vi "SG_changeFrequency.vi"(7 "MHz":i32, 8 "error in":errorcluster, 11 "VISA in":refnum<visa-resource-name>) -> (0 "error out":errorcluster, 2 "SG_Resp":string, 3 "VISA out":refnum<visa-resource-name>)   [LabVIEW 2023, in "Keysight.lvlib"]
uses:
  Keysight.lvlib
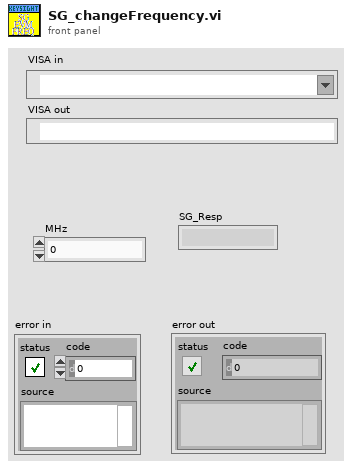
[diagram p1: front panel]
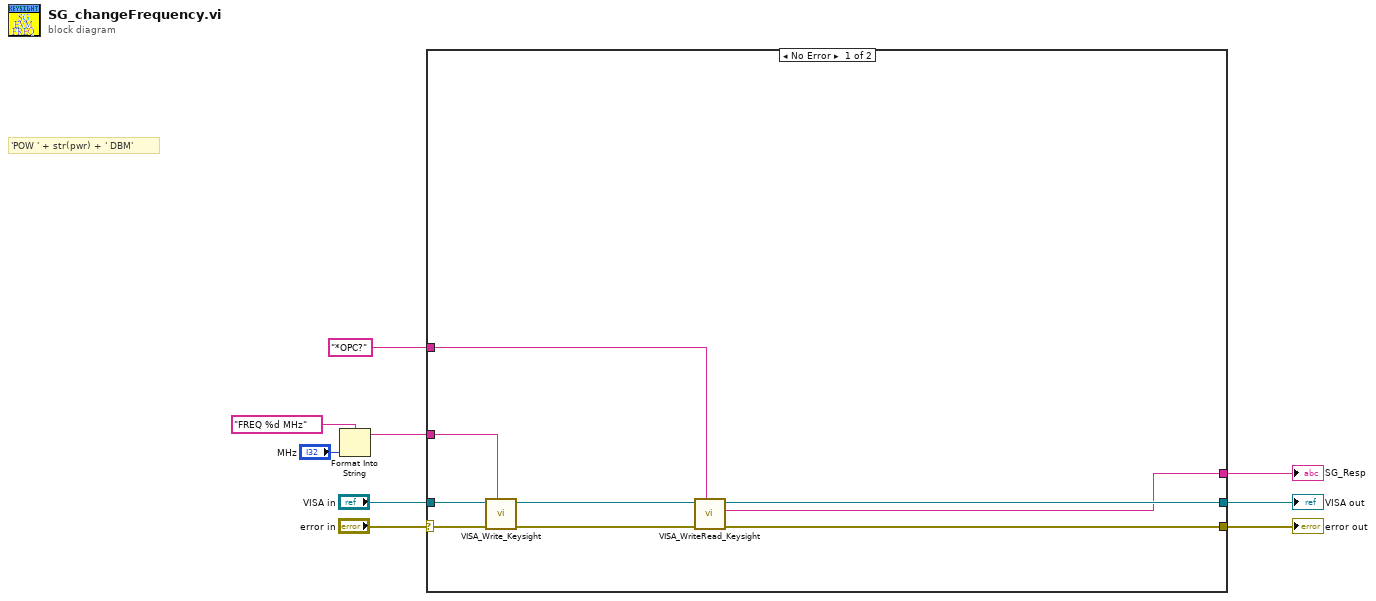
[diagram p0: block diagram]
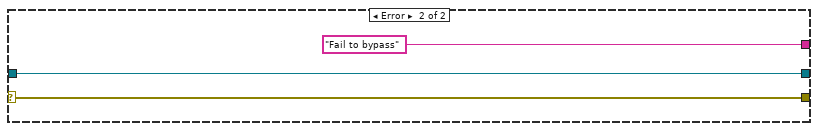
[diagram p2: hidden frame]
diagram:
  # "'POW ' + str(pwr) + ' DBM'"
  n1 = Format Into String(format string="FREQ %d MHz", "MHz") -> (resulting string=w1:string)  [unwired: 2 in, 1 out]
  n2 = case shown="No Error" "error in" {
    selector: "error in" -> [w18 w20]
    tunnel: "VISA in" -> [w17 w21]
    tunnel: w1 -> [w16 _]
    tunnel: [w15 w20] -> w7
    tunnel: [w14 w21] -> w8
    tunnel: [w13 "Fail to bypass" ("Response")] -> w9
    tunnel: "*OPC?" ("write buffer") -> [w10 _]
    frame No Error {
      n3 = call "VISA_Write_Keysight.vi"("VISA CMD"=w16, "error in"=w18, "VISA in"=w17) -> ("error out"=w11:errorcluster, "VISA out"=w12:refnum<visa-resource-name>)  [unwired: 7 in]
      n4 = call "VISA_WriteRead_Keysight.vi"("VISA_CMD"=w10, "error in"=w11, "VISA in"=w12) -> ("error out"=w15:errorcluster, "Response"=w13:string, "VISA out"=w14:refnum<visa-resource-name>)  [unwired: 6 in]
    }
    frame Error {
    }
  }
  "SG_Resp" <- w9
  "VISA out" <- w8
  "error out" <- w7
